vi "create imaq references.vi"(8 "error in (no error)":errorcluster, 11 "Thorcam in":refnum<class "Thorcam.lvclass">) -> (0 "error out":errorcluster, 3 "Thorcam out":refnum<class "Thorcam.lvclass">)   [LabVIEW 2012, in "Thorcam.lvclass"]
uses:
  Thorcam.lvclass
  Thorcam.lvclass/Thorcam.ctl
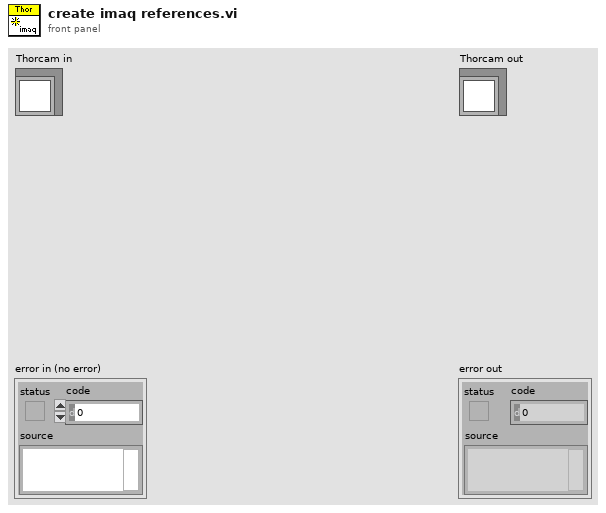
[diagram p1: front panel]
types:
  T1 = typedef "Image Type" = u32
  T2 = typedef "IMAQ Image.ctl" = refnum<image>
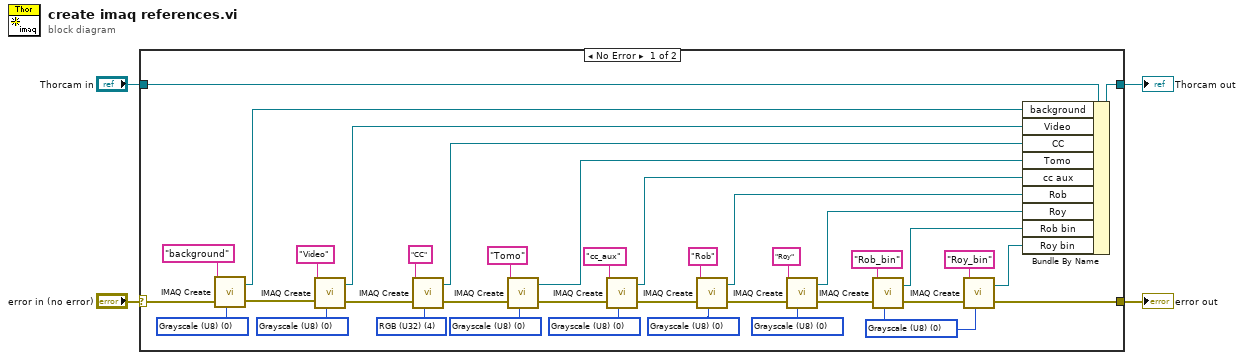
[diagram p0: block diagram]
diagram:
  n1 = case shown="No Error" "error in (no error)" {
    selector: "error in (no error)" -> [w15 w44]
    tunnel: [w10 w44] -> w3
    tunnel: [w36 w43] -> w1
    tunnel: "Thorcam in" -> [w37 w43]
    frame No Error {
      w9 = T1 0 items=["Grayscale (U8)", "Grayscale (I16)", "Grayscale (SGL)", "Complex (CSG)", "RGB (U32)", "HSL (U32)", "RGB (U64)", "Grayscale (U16)"] ("Image Type")
      w16 = T1 0 items=["Grayscale (U8)", "Grayscale (I16)", "Grayscale (SGL)", "Complex (CSG)", "RGB (U32)", "HSL (U32)", "RGB (U64)", "Grayscale (U16)"] ("Image Type")
      w21 = T1 0 items=["Grayscale (U8)", "Grayscale (I16)", "Grayscale (SGL)", "Complex (CSG)", "RGB (U32)", "HSL (U32)", "RGB (U64)", "Grayscale (U16)"] ("Image Type")
      w25 = T1 4 items=["Grayscale (U8)", "Grayscale (I16)", "Grayscale (SGL)", "Complex (CSG)", "RGB (U32)", "HSL (U32)", "RGB (U64)", "Grayscale (U16)"] ("Image Type")
      w24 = T1 0 items=["Grayscale (U8)", "Grayscale (I16)", "Grayscale (SGL)", "Complex (CSG)", "RGB (U32)", "HSL (U32)", "RGB (U64)", "Grayscale (U16)"] ("Image Type")
      w33 = T1 0 items=["Grayscale (U8)", "Grayscale (I16)", "Grayscale (SGL)", "Complex (CSG)", "RGB (U32)", "HSL (U32)", "RGB (U64)", "Grayscale (U16)"] ("Image Type")
      w34 = T1 0 items=["Grayscale (U8)", "Grayscale (I16)", "Grayscale (SGL)", "Complex (CSG)", "RGB (U32)", "HSL (U32)", "RGB (U64)", "Grayscale (U16)"] ("Image Type")
      w35 = T1 0 items=["Grayscale (U8)", "Grayscale (I16)", "Grayscale (SGL)", "Complex (CSG)", "RGB (U32)", "HSL (U32)", "RGB (U64)", "Grayscale (U16)"] ("Image Type")
      n2 = call "IMAQ Create"("Image Name"="background", "Image Type"=w16, "error in (no error)"=w15) -> ("New Image"=w13:T2, "error out"=w14:errorcluster)  [unwired: 2 in]
      n3 = call "IMAQ Create"("Image Name"="Video", "Image Type"=w21, "error in (no error)"=w14) -> ("New Image"=w18:T2, "error out"=w19:errorcluster)  [unwired: 2 in]
      n4 = call "IMAQ Create"("Image Name"="CC", "Image Type"=w25, "error in (no error)"=w19) -> ("New Image"=w22:T2, "error out"=w27:errorcluster)  [unwired: 2 in]
      n5 = call "IMAQ Create"("Image Name"="Tomo", "Image Type"=w24, "error in (no error)"=w27) -> ("New Image"=w23:T2, "error out"=w26:errorcluster)  [unwired: 2 in]
      n6 = call "IMAQ Create"("Image Name"="cc_aux", "Image Type"=w35, "error in (no error)"=w26) -> ("New Image"=w32:T2, "error out"=w42:errorcluster)  [unwired: 2 in]
      n7 = call "IMAQ Create"("Image Name"="Rob", "Image Type"=w34, "error in (no error)"=w42) -> ("New Image"=w31:T2, "error out"=w41:errorcluster)  [unwired: 2 in]
      n8 = call "IMAQ Create"("Image Name"="Roy", "Image Type"=w33, "error in (no error)"=w41) -> ("New Image"=w30:T2, "error out"=w11:errorcluster)  [unwired: 2 in]
      n9 = call "IMAQ Create"("Image Name"="Rob_bin", "Image Type"=w9, "error in (no error)"=w11) -> ("New Image"=w6:T2, "error out"=w12:errorcluster)  [unwired: 2 in]
      n10 = call "IMAQ Create"("Image Name"="Roy_bin", "Image Type"=w9, "error in (no error)"=w12) -> ("New Image"=w5:T2, "error out"=w10:errorcluster)  [unwired: 2 in]
      n11 = Bundle By Name(cluster=w37, "background"=w13, "Video"=w18, "CC"=w22, "Tomo"=w23, "cc aux"=w32, "Rob"=w31, "Roy"=w30, "Rob bin"=w6, "Roy bin"=w5) -> (w36:refnum<class "Thorcam.lvclass">)
    }
    frame Error {
    }
  }
  "error out" <- w3
  "Thorcam out" <- w1
